vi "Omniax_mDrive_Xonly_2017APXNoBK.vi"() -> ()   [LabVIEW 2015]
uses:
  <vilib>/Utility/file.llb/Read From Spreadsheet File (I64).vi
  <vilib>/Instr/_visa.llb/VISA Configure Serial Port (Instr).vi
  <userlib>/caLab/Private/Get_PV.vi
  Omniax_mDrive_GNDGlobal.vi
  <userlib>/caLab/Private/Put_DBL_PV.vi
  <vilib>/Utility/file.llb/Write To Spreadsheet File (I64).vi
  <vilib>/Utility/file.llb/Read From Spreadsheet File (string).vi
  <vilib>/Utility/file.llb/Write To Spreadsheet File (DBL).vi
panel:
  out "read buffer":string
  in  "APX:MX_RQ":dbl min=-1.5 max=1.5
  in  "APX:MX_VLC_RQ":dbl min=0.0 max=0.1 step=0.01
  out "PR P":string
  in  "X Velocity SP step/sec":i32 min=1 max=12800
  in  "X Step SP":i32=-20000 min=-2304000 max=2304000 step=500
  out "X Step PV":i32 max=2000
  out "Boolean 2":bool
  out "R Velocity MVdeg/sec":dbl format="%.3f"
  out "R Position MV deg":dbl
  out "Z Velocity MV mm/sec":dbl format="%.3f"
  out "Z Position MV mm":dbl
  out "Y Velocity MV mm/sec":dbl format="%.3f"
  out "Y Position MV mm":dbl
  out "X Velocity MV mm/sec":dbl format="%.3f"
  out "X Position MV mm":dbl
  out "Presets":i32[][](array[numeric])
  in  "stop":bool
  in  "Tab Control 3":enum32{"Status", "Reset"}(tab)
  out "APX:X_LIM":bool
  out "APX:MX_MVG":bool
  out "APX:MX_RDY":bool
  out "sample NC":bool
  out "Z<350?":bool
  in  "Reset X Position mm":dbl
  out "Reset X Motor Steps":i32
  in  "Reset":bool
  out "R Backlash steps/sec":i32
  out "R Backlash":i32
  out "R Holding Current %":i32
  out "R Run Current %":i32
  out "R offset deg":dbl
  out "R deg/rev":dbl
  out "R steps/rev":u32
  out "R velocity PV step/sec":i32
  out "Z Backlash steps/sec":i32
  out "Z Backlash":i32
  out "Z Holding Current %":i32
  out "Z Run Current %":i32
  out "Z offset mm":dbl
  out "Z mm/rev":dbl
  out "Z steps/rev":u32
  out "Z  velocity PV step/sec":i32
  out "APX:MX_PV":dbl
  out "X velocity PV step/sec":i32
  out "X Backlash steps/sec":i32
  out "X Backlash":i32
  out "X Holding Current %":i32
  out "X Run Current %":i32
  out "X offset mm":dbl
  out "X mm/rev":dbl
  out "X steps/rev":u32
  out "X MAXPOS":i32=-34296
  out "X MINPOS":i32=-94296
  out "X COM PORT":refnum<visa-resource-name>="COM5"
  out "Y Backlash steps/sec":i32
  out "Y Backlash":i32
  out "Y Holding Current %":i32
  out "Y Run Current %":i32
  out "Y offset mm":dbl
  out "Y mm/rev":dbl
  out "Y steps/rev":u32
  out "Y velocity PV step/sec":i32
  in  "APX:MXYZR_STOP":bool
  # "APX:MX"
  # "Goto position"
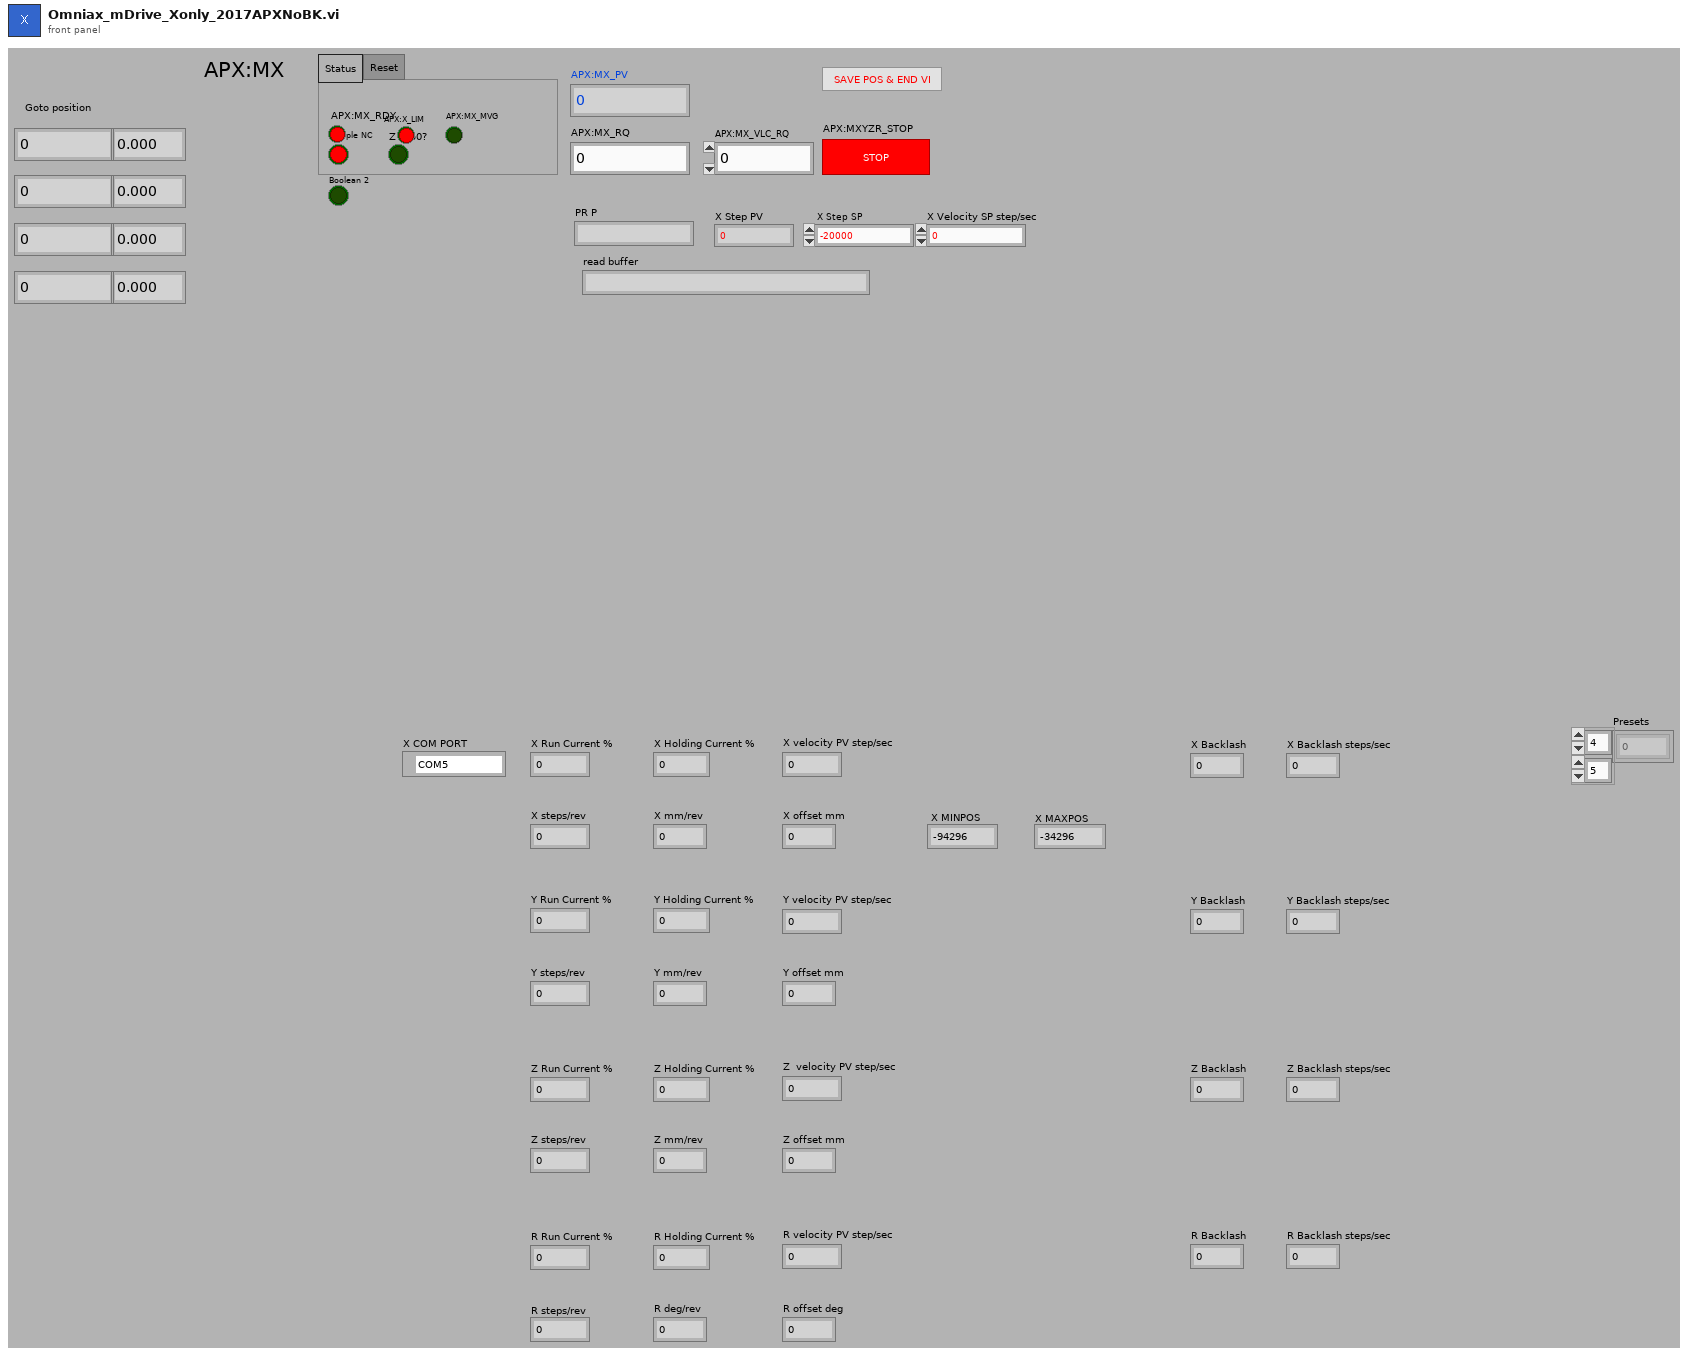
[diagram p1: front panel]
types:
  T1 = enum16{"Stop", "Reset", "Run Current", "Holding Current", "Accel Rate", "Decel Rate", "Move to Relative Position", "Move to Absolute Position", "Echo Mode", "Print Parameter", "Send String", "Microstep Resolution", "Set Current Position", "Max Velocity"}
  T2 = enum8{"Enabled", "Disabled", "Disabled and Grayed Out"}
  T3 = cluster{"first row[0]":i64, "first row[1]":i64, "first row[2]":i64, "first row[3]":i64, "first row[4]":i64, "first row[5]":i64, "first row[6]":i64, "first row[7]":i64, "first row[8]":i64}
  T4 = cluster{"Value[0]":i32, "Value[1]":i32, "Value[2]":i32, "Value[3]":i32, "Value[4]":i32, "Value[5]":i32, "Value[6]":i32, "Value[7]":i32, "Value[8]":i32}
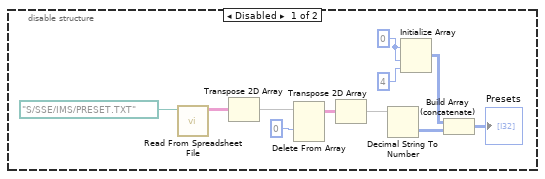
[diagram p2: hidden frame]
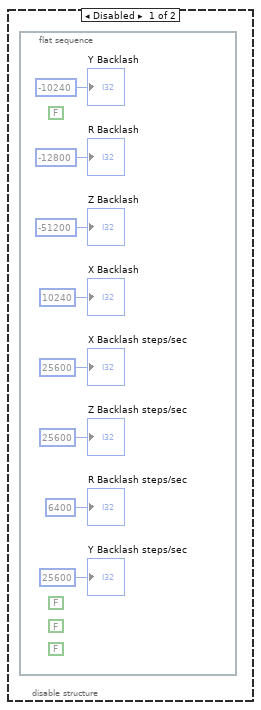
[diagram p3: hidden frame]
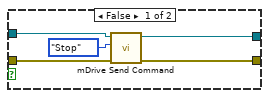
[diagram p9: hidden frame]
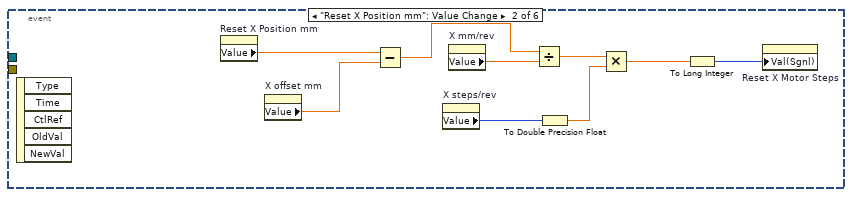
[diagram p14: hidden frame]
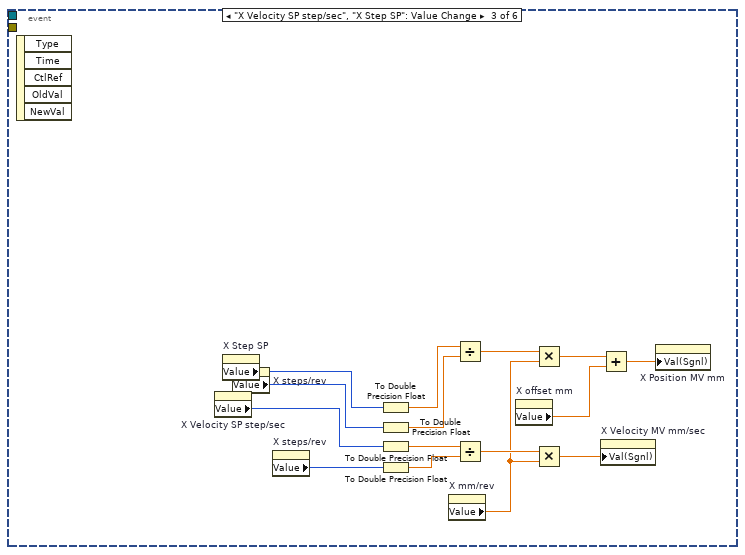
[diagram p15: hidden frame]
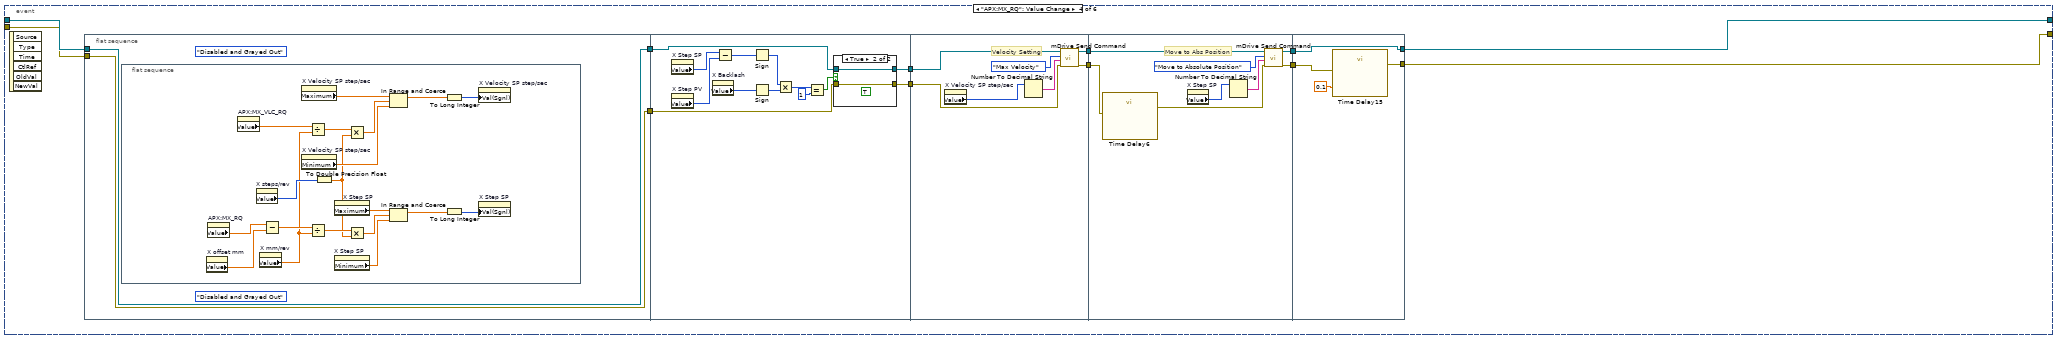
[diagram p16: hidden frame]
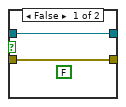
[diagram p17: hidden frame]
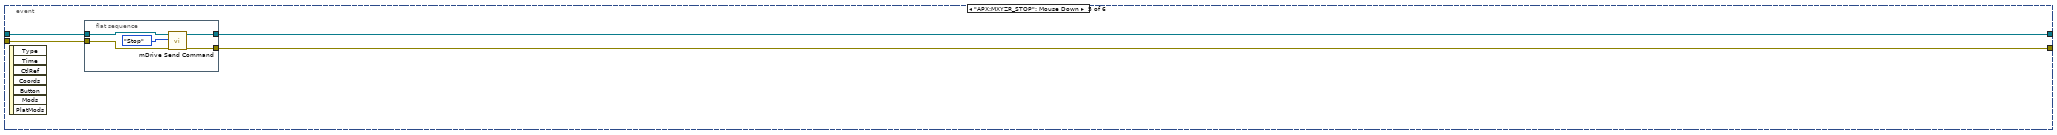
[diagram p18: hidden frame]
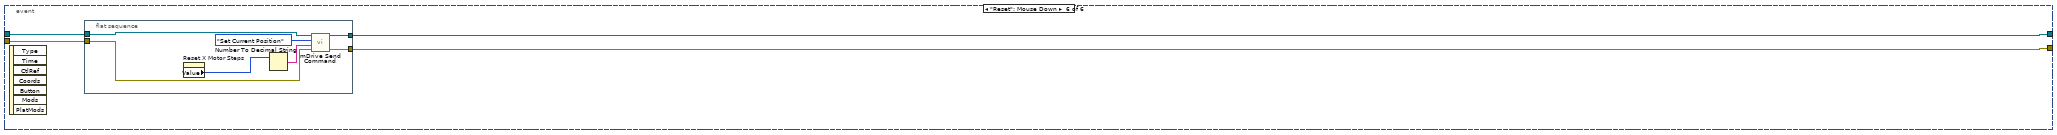
[diagram p19: hidden frame]
diagram:
  n1 = flat-sequence {
    tunnel: [w27] -> w9
    tunnel: [w26] -> w8
    tunnel: [w37] -> w12
    tunnel: w9 -> [w43]
    tunnel: w8 -> [w44]
    tunnel: [w38] -> w2
    tunnel: [w36] -> w1
    tunnel: w12 -> [_]
    tunnel: [w48] -> w11
    tunnel: [w51] -> w10
    tunnel: w2 -> [w49]
    tunnel: w1 -> [w47]
    tunnel: [w60] -> w25
    tunnel: [w62] -> w24
    tunnel: w11 -> [w61]
    tunnel: w10 -> [w63]
    tunnel: w25 -> [w70]
    tunnel: [w69] -> w23
    tunnel: w24 -> [w67]
    tunnel: [w68] -> w22
    tunnel: [w80] -> w21
    tunnel: [w81] -> w20
    tunnel: w23 -> [w79]
    tunnel: w22 -> [w78]
    tunnel: w21 -> [w91]
    tunnel: w20 -> [w90]
    tunnel: [w93] -> w15
    tunnel: [w92] -> w14
    tunnel: [w87] -> w13
    tunnel: [w98] -> w18
    tunnel: [w99] -> w19
    tunnel: w15 -> [w99]
    tunnel: w14 -> [w98]
    tunnel: w13 -> [w94]
    frame #0 {
      w34 = refnum<visa-resource-name> "COM12" ("COM PORT")
      w32 = u16 0 items=["None", "XON/XOFF", "RTS/CTS", "XON/XOFF & RTS/CTS", "DTR/DSR", "XON/XOFF & DTR/DSR"] ("flow control (0:none)")
      w31 = u16 10 items=["1.0"=10, "1.5"=15, "2.0"=20] ("stop bits (10: 1 bit)")
      # "Stop bits"
      n2 = call-poly "VISA Configure Serial Port"("VISA resource name"=w34, "timeout (10sec)"=u32 10000, "baud rate (9600)"=u32 9600, "data bits (8)"=u16 8, "parity (0:none)"=enum16{"None", "Odd", "Even", "Mark", "Space"}."None", "stop bits (10: 1 bit)"=w31, "flow control (0:none)"=w32) -> ("VISA resource name out"=w27:refnum<visa-resource-name>, "error out"=w26:errorcluster)  [unwired: 7 in]
      "X COM PORT" <- w34
    }
    frame #1 {
      n3 = VISA Flush I/O Buffer(VISA resource name=w43) -> (VISA resource name out=w42:refnum<visa-resource-name>)  [unwired: 2 in, 1 out]
      n4 = call "mDrive Send Command.vi"("error in (no error)"=w44, "Extra"="EM 2", "Command"=T1."Send String", "VISA resource name"=w42) -> ("error out"=w39:errorcluster, "VISA resource name out"=w37:refnum<visa-resource-name>)  [unwired: 3 in, 1 out]
      n5 = call "mDrive Send Command.vi"("error in (no error)"=w39, "Extra"="PR EE", "Command"=T1."Send String", "VISA resource name"=w37) -> ("error out"=w38:errorcluster, "read buffer"=→"read buffer":string, "VISA resource name out"=w36:refnum<visa-resource-name>)  [unwired: 3 in]
    }
    frame #2 {
      n6 = Number To Decimal String(number=1000000) -> (decimal integer string=w52:string)  [unwired: 1 in]
      n7 = call "mDrive Send Command.vi"("error in (no error)"=w49, "Extra"=w52, "Command"=T1."Accel Rate", "VISA resource name"=w47) -> ("error out"=w50:errorcluster, "VISA resource name out"=w56:refnum<visa-resource-name>)  [unwired: 3 in, 1 out]
      n8 = call "mDrive Send Command.vi"("error in (no error)"=w50, "Extra"=w52, "Command"=T1."Decel Rate", "VISA resource name"=w56) -> ("error out"=w51:errorcluster, "VISA resource name out"=w48:refnum<visa-resource-name>)  [unwired: 3 in, 1 out]
    }
    frame #3 {
      # "Run Current %"
      n9 = property on="X Run Current %" class="DigNum (strict)"() -> ("Value"=w58:i32)  [unwired: 2 in, 2 out]
      n10 = Number To Decimal String(number=w58) -> (decimal integer string=w59:string)  [unwired: 1 in]
      n11 = call "mDrive Send Command.vi"("error in (no error)"=w63, "Extra"=w59, "Command"=T1."Run Current", "VISA resource name"=w61) -> ("error out"=w62:errorcluster, "VISA resource name out"=w60:refnum<visa-resource-name>)  [unwired: 3 in, 1 out]
    }
    frame #4 {
      # "Holding Current %"
      n12 = property on="X Holding Current %" class="DigNum (strict)"() -> ("Value"=w65:i32)  [unwired: 2 in, 2 out]
      n13 = Number To Decimal String(number=w65) -> (decimal integer string=w66:string)  [unwired: 1 in]
      n14 = call "mDrive Send Command.vi"("error in (no error)"=w67, "Extra"=w66, "Command"=T1."Holding Current", "VISA resource name"=w70) -> ("error out"=w68:errorcluster, "VISA resource name out"=w69:refnum<visa-resource-name>)  [unwired: 3 in, 1 out]
    }
    frame #5 {
      # "Velocity Max"
      n15 = property on="X Velocity SP step/sec" class="DigNum (strict)"() -> ("Value"=w77:i32)  [unwired: 2 in, 2 out]
      n16 = Number To Decimal String(number=w77) -> (decimal integer string=w76:string)  [unwired: 1 in]
      n17 = call "mDrive Send Command.vi"("error in (no error)"=w78, "Extra"=w76, "Command"=T1."Max Velocity", "VISA resource name"=w79) -> ("error out"=w74:errorcluster, "VISA resource name out"=w84:refnum<visa-resource-name>)  [unwired: 3 in, 1 out]
      n18 = call "mDrive Send Command.vi"("error in (no error)"=w74, "Extra"="VM", "Command"=T1."Print Parameter", "VISA resource name"=w84) -> ("error out"=w81:errorcluster, "read buffer"=w82:string, "VISA resource name out"=w80:refnum<visa-resource-name>)  [unwired: 3 in]
      n19 = Decimal String To Number(string=w82, offset=0) -> (number=w75:i32)  [unwired: 1 in, 1 out]
      n20 = property on="X velocity PV step/sec" class="DigNum (strict)"("Val(Sgnl)"=w75) -> ()  [unwired: 2 in, 2 out]
    }
    frame #6 {
      # "PRINT POSITION"
      n21 = call "mDrive Send Command.vi"("error in (no error)"=w90, "Extra"="P", "Command"=T1."Print Parameter", "VISA resource name"=w91) -> ("error out"=w92:errorcluster, "read buffer"=w89:string, "VISA resource name out"=w93:refnum<visa-resource-name>)  [unwired: 3 in]
      n22 = Decimal String To Number(string=w89, offset=0) -> (number=w87:i32)  [unwired: 1 in, 1 out]
    }
    frame #7 {
      w96 = -2304000 ("lower limit")
      w97 = 2304000 ("upper limit")
      n23 = property on="X Step SP" class="DigNum (strict)"("Val(Sgnl)"=w94) -> ()  [unwired: 2 in, 2 out]
      n24 = property on="X Step SP" class="DigNum (strict)"("Maximum"=w97) -> ()  [unwired: 2 in, 2 out]
      n25 = In Range and Coerce(upper limit=w97, x=w94, lower limit=w96) -> (In Range?=w95:bool)  [unwired: 1 out]
      n26 = property on="X Step SP" class="DigNum (strict)"("Minimum"=w96) -> ()  [unwired: 2 in, 2 out]
      n27 = property on="APX:X_LIM" class="Bool (strict)"("Val(Sgnl)"=w95) -> ()  [unwired: 2 in, 2 out]
      "X MINPOS" <- w96
      "X MAXPOS" <- w97
    }
  }
  n28 = disable-structure shown="Enabled" {
    frame Disabled {
      w100 = 0 ("dimension size")
      n29 = call-poly <vilib>:"Read From Spreadsheet File.vi"("file path (dialog if empty)"=path "S:/SSE/IMS/PRESET.TXT") -> ("all rows"=w106:string[][])  [unwired: 6 in, 4 out]
      n30 = Transpose 2D Array(2D array=w106) -> (transposed array=w107:string[][])
      n31 = Delete From Array(array=w107, index (row)=0) -> (deleted portion=w108:string[], array with subset deleted=w110:string[][])  [unwired: 2 in]
      n32 = Transpose 2D Array(2D array=w110) -> (transposed array=w111:string[][])
      n33 = Decimal String To Number(string=w111) -> (number=w109:i32[][])  [unwired: 2 in, 1 out]
      n34 = Initialize Array(w100, w100, 4 ("dimension size")) -> (w103:i32[][])
      n35 = Build Array (concatenate)(w103, w109) -> (→"Presets":i32[][])
    }
    frame Enabled {
    }
  }
  n36 = flat-sequence {
    frame #0 {
      (unwired) 1.0 ("Data Entry Limits:Minimum")
      w115 = -3.0 ("R deg/rev")
      w113 = u32 51200 ("step/rev")
      n37 = To Double Precision Float(number=w113) -> (double precision float=w114:dbl)
      n38 = To Double Precision Float(number=10000 ("Value (Signaling)")) -> (double precision float=w119:dbl)
      n39 = Divide(x=w119, y=w114) -> (x/y=w118:dbl)
      n40 = Multiply(x=w118, y=w115) -> (x*y=w116:dbl)
      n41 = Absolute Value(x=w116) -> ()  [unwired: 1 out]
      "R offset deg" <- 0.0 ("R offset deg")
      "R deg/rev" <- w115
      "R steps/rev" <- w113
    }
  }
  n42 = flat-sequence {
    frame #0 {
      w121 = 0.2 ("Z mm/rev")
      w120 = u32 51200 ("step/rev")
      (unwired) 1.0 ("Data Entry Limits:Minimum")
      n43 = To Double Precision Float(number=204800 ("Value (Signaling)")) -> (double precision float=w125:dbl)
      n44 = To Double Precision Float(number=w120) -> (double precision float=w124:dbl)
      n45 = Divide(x=w125, y=w124) -> (x/y=w123:dbl)
      n46 = Multiply(x=w123, y=w121) -> ()  [unwired: 1 out]
      "Z offset mm" <- 0.0 ("Z offset mm")
      "Z mm/rev" <- w121
      "Z steps/rev" <- w120
    }
  }
  n47 = disable-structure shown="Enabled" {
    frame Disabled {
      n48 = flat-sequence {
        frame #0 {
          w127 = FALSE ("Value (Signaling)")
          w130 = FALSE ("Value (Signaling)")
          w133 = FALSE ("Value (Signaling)")
          w134 = FALSE ("Value (Signaling)")
          "Z Backlash steps/sec" <- 25600 ("Z Backlash steps/sec")
          "Z Backlash" <- -51200 ("Z Backlash")
          "X Backlash steps/sec" <- 25600 ("Value (Signaling)")
          "X Backlash" <- 10240 ("Backlash2")
          "Y Backlash" <- -10240 ("Backlash2")
          "Y Backlash steps/sec" <- 25600 ("Value (Signaling)")
          "R Backlash steps/sec" <- 6400 ("R Backlash steps/sec")
          "R Backlash" <- -12800 ("R Backlash")
        }
      }
    }
    frame Enabled {
    }
  }
  n49 = flat-sequence {
    frame #0 {
      "Z Holding Current %" <- 20 ("Z Holding Current %")
      "Z Run Current %" <- 40 ("Z Run Current %")
      "X Run Current %" <- 40 ("Run Current %")
      "X Holding Current %" <- 20 ("Holding Current %")
      "Y Run Current %" <- 40 ("Run Current %")
      "Y Holding Current %" <- 20 ("Holding Current %")
      "R Holding Current %" <- 15 ("R Holding Current %")
      "R Run Current %" <- 80 ("R Run Current %")
    }
  }
  n50 = flat-sequence {
    frame #0 {
      (unwired) 0.1 ("Value (Signaling)")
      (unwired) FALSE ("Value (Signaling)")
      (unwired) T2."Disabled and Grayed Out" ("Disabled")
      (unwired) T2."Disabled and Grayed Out" ("Disabled")
      (unwired) 0.1 ("Value (Signaling)")
      (unwired) FALSE ("Value (Signaling)")
      (unwired) 0.1 ("Value (Signaling)")
      (unwired) FALSE ("Value (Signaling)")
      (unwired) 0.1 ("Value (Signaling)")
      (unwired) FALSE ("Value (Signaling)")
    }
  }
  n51 = flat-sequence {
    frame #0 {
      w149 = 0.2 ("MM/rev")
      w152 = u32 51200 ("step/rev")
      w147 = 12800 ("Value (Signaling)")
      # "a=1000000"
      n52 = property on="X Velocity SP step/sec" class="DigNum (strict)"("Minimum"=1.0 ("Data Entry Limits:Minimum")) -> ()  [unwired: 2 in, 2 out]
      n53 = To Double Precision Float(number=w147) -> (double precision float=w153:dbl)
      n54 = To Double Precision Float(number=w152) -> (double precision float=w151:dbl)
      n55 = property on="X Velocity SP step/sec" class="DigNum (strict)"("Val(Sgnl)"=w147) -> ()  [unwired: 2 in, 2 out]
      n56 = property on="X Velocity SP step/sec" class="DigNum (strict)"("Maximum"=w153) -> ()  [unwired: 2 in, 2 out]
      n57 = Divide(x=w153, y=w151) -> (x/y=w148:dbl)
      n58 = Multiply(x=w148, y=w149) -> (x*y=w150:dbl)
      n59 = property on="APX:MX_VLC_RQ" class="DigNum (strict)"("Val(Sgnl)"=w150) -> ()  [unwired: 2 in, 2 out]
      "X offset mm" <- 0.0 ("offset")
      "X steps/rev" <- w152
      "X mm/rev" <- w149
    }
  }
  n60 = flat-sequence {
    frame #0 {
      w158 = 0.2 ("MM/rev")
      w160 = u32 51200 ("step/rev")
      (unwired) 1.0 ("Data Entry Limits:Minimum")
      n61 = To Double Precision Float(number=128000 ("Value (Signaling)")) -> (double precision float=w161:dbl)
      n62 = To Double Precision Float(number=w160) -> (double precision float=w159:dbl)
      n63 = Divide(x=w161, y=w159) -> (x/y=w157:dbl)
      n64 = Multiply(x=w157, y=w158) -> ()  [unwired: 1 out]
      "Y offset mm" <- 0.0 ("offset")
      "Y steps/rev" <- w160
      "Y mm/rev" <- w158
    }
  }
  n65 = call-poly <vilib>:"Read From Spreadsheet File.vi"("file path (dialog if empty)"=path "S:/SSE/IMS/POSX.TXT") -> ("first row"=w6:i64[])  [unwired: 6 in, 4 out]
  n66 = Array To Cluster(array=w6) -> (cluster=w5:T3)
  n67 = Unbundle(w5) -> ("first row[0]"=w3:i64)  [unwired: 8 out]
  n68 = property on="Reset X Motor Steps" class="DigNum (strict)"("Val(Sgnl)"=w3) -> ()  [unwired: 2 in, 2 out]
  n69 = while {
    tunnel: w19 -> [w167]
    tunnel: w18 -> [w166]
    tunnel: [w165] -> w17
    tunnel: [w164] -> w16
    stop <- "stop" stop-if-true
    n70 = disable-structure shown="Disabled" {
      frame Disabled {
        n71 = case shown="True" {
          selector: _ -> [_ _]
          tunnel: _ -> [_ w194]
          frame False {
          }
          frame True {
            n72 = property on="Presets" class="Arr (strict)"() -> ("Value"=w191:i32[][])  [unwired: 2 in, 2 out]
            n73 = Index Array(array=w191, index (row)=w194) -> (element=w193:i32[])  [unwired: 1 in]
            n74 = Array To Cluster(array=w193) -> (cluster=w192:T4)
            n75 = Unbundle(w192) -> ("Value[0]"=w190:i32, "Value[1]"=w189:i32, "Value[2]"=w188:i32, "Value[3]"=w187:i32)  [unwired: 5 out]
            n76 = property on="X Step SP" class="DigNum (strict)"("Val(Sgnl)"=w190) -> ()  [unwired: 2 in, 2 out]
          }
        }
        n77 = case shown="True" w170 {
          tunnel: [_ w186] -> w171
          frame False {
          }
          frame True {
            n78 = property on="X Step PV" class="DigNum (strict)"() -> ("Value"=w181:i32)  [unwired: 2 in, 2 out]
            n79 = Build Array(w186) -> (w185:void[], w182:dbl)
            n80 = Build Array(w181) -> (w184:i32[], w180:i32, w179:i32, w178:i32)
            n81 = property on="Presets" class="Arr (strict)"() -> ("Value"=w183:i32[][])  [unwired: 2 in, 2 out]
            n82 = Build Array (concatenate)(w183, w184) -> (w177:i32[][])
            n83 = property on="Presets" class="Arr (strict)"("Val(Sgnl)"=w177) -> ()  [unwired: 2 in, 2 out]
          }
        }
        n84 = case shown="True" w169 {
          tunnel: w171 -> [_ w176]
          frame False {
          }
          frame True {
            n85 = Delete From Array(array=w176) -> (array with subset deleted=w175, index=w174:i32)  [unwired: 1 in, 1 out]
            n86 = property on="Presets" class="Arr (strict)"() -> ("Value"=w173:i32[][])  [unwired: 2 in, 2 out]
            n87 = Delete From Array(array=w173, index (row)=w174) -> (array with subset deleted=w172:i32[][])  [unwired: 2 in, 1 out]
            n88 = property on="Presets" class="Arr (strict)"("Val(Sgnl)"=w172) -> ()  [unwired: 2 in, 2 out]
          }
        }
      }
      frame Enabled {
      }
    }
    n89 = event shown="[0] Timeout" {
      selector: _ -> [_ _ _ _ _ _]
      dyn-events: _ -> [_ _ _ _ _ _]
      timeout: 100 -> [_ _ _ _ _ _]
      tunnel: w167 -> [w207 _ _ w393 w460 w471]
      tunnel: w166 -> [w205 _ _ w392 w459 w470]
      tunnel: [w209 _ _ w391 w462 w469] -> w165
      tunnel: [w208 _ _ w390 w461 w468] -> w164
      event Timeout {
        n90 = event-data() -> ()  [unwired: 1 in, 2 out]
        n91 = flat-sequence {
          tunnel: [w265] -> w220
          tunnel: [w243] -> w219
          tunnel: [w254] -> w218
          tunnel: [w234] -> w217
          tunnel: w206 -> [w233]
          tunnel: w204 -> [w232]
          tunnel: [w228] -> w203
          tunnel: w220 -> [w277]
          tunnel: [w277] -> w216
          tunnel: w219 -> [w276]
          tunnel: [w276] -> w215
          tunnel: w218 -> [w275]
          tunnel: [w275] -> w214
          tunnel: w217 -> [w274]
          tunnel: [w274] -> w213
          tunnel: w203 -> [w273]
          tunnel: [w273] -> w201
          tunnel: w216 -> [w281]
          tunnel: [w282] -> w212
          tunnel: w215 -> [w284]
          tunnel: [w283] -> w211
          tunnel: w214 -> [w280]
          tunnel: [w279] -> w210
          tunnel: w213 -> [w279]
          tunnel: [w278] -> w202
          tunnel: w201 -> [w278]
          tunnel: w212 -> [w296]
          tunnel: w211 -> [w297]
          tunnel: w210 -> [w298]
          tunnel: [w295] -> w208
          tunnel: [w294] -> w209
          tunnel: w202 -> [w292]
          frame #0 {
            w238 = 0.1 ("Delay Time (s)")
            n92 = call "mDrive Send Command.vi"("error in (no error)"=w232, "Extra"="P", "Command"=T1."Print Parameter", "VISA resource name"=w233) -> ("error out"=w260:errorcluster, "read buffer"=w264:string, "VISA resource name out"=w262:refnum<visa-resource-name>)  [unwired: 3 in]
            "PR P" <- w264
            n93 = call "Time Delay12"("error in (no error)"=w260, "Delay Time (s)"=w238) -> ("error out"=w259:errorcluster)  [unwired: 9 in]
            n94 = Decimal String To Number(string=w264, offset=0) -> (number=w245:i32)  [unwired: 1 in, 1 out]
            n95 = property on="X Step SP" class="DigNum (strict)"() -> ("Maximum"=w256:dbl)  [unwired: 2 in, 2 out]
            n96 = property on="X Step SP" class="DigNum (strict)"() -> ("Minimum"=w258:dbl)  [unwired: 2 in, 2 out]
            n97 = To Long Integer(number=w245) -> (32bit integer=w246:i32)
            n98 = property on="X steps/rev" class="DigNum (strict)"() -> ("Value"=w252:u32)  [unwired: 2 in, 2 out]
            n99 = property on="X Step PV" class="DigNum (strict)"("Val(Sgnl)"=w246) -> ()  [unwired: 2 in, 2 out]
            n100 = disable-structure shown="Disabled" {
              disable-tunnel: [w272 _] -> w265
              disable-tunnel: w262 -> [w271 _]
              disable-tunnel: [w270 _] -> w261
              disable-tunnel: w259 -> [w269 _]
              disable-tunnel: T1."Print Parameter" ("Command") -> [w268 _]
              disable-tunnel: "MV" ("Extra") -> [w267 _]
              disable-tunnel: [w266 _] -> w231
              frame Disabled {
                n101 = call "mDrive Send Command.vi"("error in (no error)"=w269, "Extra"=w267, "Command"=w268, "VISA resource name"=w271) -> ("error out"=w270:errorcluster, "read buffer"=w266:string, "VISA resource name out"=w272:refnum<visa-resource-name>)  [unwired: 3 in]
              }
              frame Enabled {
              }
            }
            n102 = To Long Integer(number=w256) -> (32bit integer=w255:i32)
            n103 = To Long Integer(number=w258) -> (32bit integer=w257:i32)
            n104 = In Range and Coerce(upper limit=w255, x=w246, lower limit=w257) -> (In Range?=w254:bool)  [unwired: 1 out]
            n105 = To Double Precision Float(number=w246) -> (double precision float=w247:dbl)
            n106 = To Double Precision Float(number=w252) -> (double precision float=w253:dbl)
            n107 = property on="APX:X_LIM" class="Bool (strict)"("Val(Sgnl)"=w254) -> ()  [unwired: 2 in, 2 out]
            n108 = Divide(x=w247, y=w253) -> (x/y=w251:dbl)
            n109 = call "Time Delay11"("error in (no error)"=w261, "Delay Time (s)"=w238) -> ("error out"=w243:errorcluster)  [unwired: 9 in]
            n110 = Decimal String To Number(string=w231, offset=0 ("offset (0)")) -> (number=w237:i32)  [unwired: 1 in, 1 out]
            n111 = Not Equal?(x=w231, y="") -> (x != y?=w229:bool)
            n112 = property on="X mm/rev" class="DigNum (strict)"() -> ("Value"=w250:dbl)  [unwired: 2 in, 2 out]
            n113 = property on="X offset mm" class="DigNum (strict)"() -> ("Value"=w248:dbl)  [unwired: 2 in, 2 out]
            n114 = Multiply(x=w251, y=w250) -> (x*y=w249:dbl)
            n115 = Number To Boolean Array(number=w237) -> (Boolean array=w236:bool[])
            n116 = property on="APX:MX_RDY" class="Bool (strict)"("Val(Sgnl)"=w229) -> ()  [unwired: 2 in, 2 out]
            n117 = Add(x=w249, y=w248) -> (x+y=w228:dbl)
            n118 = Index Array(array=w236, index=0) -> (element=w234:bool)
            n119 = property on="APX:MX_PV" class="DigNum (strict)"("Val(Sgnl)"=w228) -> ()  [unwired: 2 in, 2 out]
            n120 = property on="APX:MX_MVG" class="Bool (strict)"("Val(Sgnl)"=w234) -> ()  [unwired: 2 in, 2 out]
          }
          frame #1 {
          }
          frame #2 {
            n121 = case shown="False" w280 {
              tunnel: w281 -> [w287 w291]
              tunnel: [w288 w291] -> w282
              tunnel: [w289 w290] -> w283
              tunnel: w284 -> [w286 w290]
              frame False {
                n122 = call "mDrive Send Command.vi"("error in (no error)"=w286, "Command"=T1."Stop", "VISA resource name"=w287) -> ("error out"=w289:errorcluster, "VISA resource name out"=w288:refnum<visa-resource-name>)  [unwired: 4 in, 1 out]
              }
              frame True {
              }
            }
            "Boolean 2" <- w280
          }
          frame #3 {
            n123 = disable-structure shown="Disabled" {
              disable-tunnel: w298 -> [w304 _]
              disable-tunnel: w297 -> [w302 _]
              disable-tunnel: w296 -> [w301 _]
              disable-tunnel: [w300 _] -> w295
              disable-tunnel: [w299 _] -> w294
              frame Disabled {
                n124 = Implies(1:w304) -> (0:w303:bool, 2:w305:bool)
                n125 = case shown="False" w303 {
                  tunnel: w302 -> [w312 w364]
                  tunnel: w301 -> [w311 w365]
                  tunnel: [w310 w364] -> w300
                  tunnel: [w309 w365] -> w299
                  frame False {
                    # "Backlash"
                    n126 = flat-sequence {
                      tunnel: [w327] -> w324
                      tunnel: [w329] -> w323
                      tunnel: [w328] -> w322
                      tunnel: w312 -> [w326]
                      tunnel: w311 -> [w325]
                      tunnel: w324 -> [w337]
                      tunnel: [w337] -> w321
                      tunnel: w323 -> [w336]
                      tunnel: w322 -> [w335]
                      tunnel: [w334] -> w320
                      tunnel: [w333] -> w319
                      tunnel: [w332] -> w308
                      tunnel: w321 -> [w347]
                      tunnel: w320 -> [w346]
                      tunnel: w319 -> [w344]
                      tunnel: [w345] -> w318
                      tunnel: [w344] -> w317
                      tunnel: [w343] -> w314
                      tunnel: [w342] -> w313
                      tunnel: w308 -> [w342]
                      tunnel: w318 -> [w358]
                      tunnel: w317 -> [w351]
                      tunnel: [w358] -> w316
                      tunnel: [w357] -> w315
                      tunnel: w314 -> [w357]
                      tunnel: w313 -> [w353]
                      tunnel: [w352] -> w306
                      tunnel: w316 -> [w362]
                      tunnel: w315 -> [w361]
                      tunnel: [w360] -> w310
                      tunnel: [w359] -> w307
                      tunnel: w306 -> [w359]
                      tunnel: [w363] -> w309
                      tunnel: w307 -> [w363]
                      frame #0 {
                        n127 = property on="X Backlash steps/sec" class="DigNum (strict)"() -> ("Value"=w327:i32)  [unwired: 2 in, 2 out]
                        n128 = Number To Decimal String(number=w327) -> (decimal integer string=w330:string)  [unwired: 1 in]
                        n129 = call "mDrive Send Command.vi"("error in (no error)"=w326, "Extra"=w330, "Command"=T1."Max Velocity", "VISA resource name"=w325) -> ("error out"=w328:errorcluster, "VISA resource name out"=w329:refnum<visa-resource-name>)  [unwired: 3 in, 1 out]
                      }
                      frame #1 {
                        n130 = property on="X Backlash" class="DigNum (strict)"() -> ("Value"=w332:i32)  [unwired: 2 in, 2 out]
                        n131 = Number To Decimal String(number=w332) -> (decimal integer string=w338:string)  [unwired: 1 in]
                        n132 = call "mDrive Send Command.vi"("error in (no error)"=w335, "Extra"=w338, "Command"=T1."Move to Relative Position", "VISA resource name"=w336) -> ("error out"=w334:errorcluster, "VISA resource name out"=w333:refnum<visa-resource-name>)  [unwired: 3 in, 1 out]
                      }
                      frame #2 {
                        n133 = To Double Precision Float(number=w342) -> (double precision float=w340:dbl)
                        n134 = To Double Precision Float(number=w347) -> (double precision float=w349:dbl)
                        n135 = Absolute Value(x=w340) -> (abs(x)=w341:dbl)
                        n136 = Divide(x=w341, y=w349) -> (x/y=w350:dbl)
                        n137 = Add(x=w350, y=0.3) -> (x+y=w343:dbl)
                        n138 = call "Time Delay13"("error in (no error)"=w346, "Delay Time (s)"=w343) -> ("error out"=w345:errorcluster)  [unwired: 9 in]
                      }
                      frame #3 {
                        n139 = Negate(x=w353) -> (-x=w354:i32)
                        n140 = Number To Decimal String(number=w354) -> (decimal integer string=w355:string)  [unwired: 1 in]
                        n141 = call "mDrive Send Command.vi"("Extra"=w355, "Command"=T1."Move to Relative Position", "VISA resource name"=w351) -> ("VISA resource name out"=w352:refnum<visa-resource-name>)  [unwired: 4 in, 2 out]
                      }
                      frame #4 {
                        n142 = call "Time Delay14"("error in (no error)"=w362, "Delay Time (s)"=w361) -> ("error out"=w360:errorcluster)  [unwired: 9 in]
                      }
                      frame #5 {
                        (unwired) FALSE ("Value (Signaling)")
                      }
                    }
                  }
                  frame True {
                  }
                }
              }
              frame Enabled {
              }
            }
            n143 = call-poly <userlib>:"CaLabPut.vi"("Value"=w292, "PV Name"="APX:OmniaxX") -> ()  [unwired: 6 in, 4 out]
          }
        }
        n144 = call-poly "CaLabGet.vi"("PV Name"="APX:OmniaxZ") -> ("1rst Value (number)"=w199:dbl)  [unwired: 8 in, 6 out]
        n145 = Less?(x=w199, y=349.0) -> (x < y?=w195:bool)
        "Z<350?" <- w195
        n146 = global read "Omniax_mDrive_GNDGlobal.vi" "sample NC"() -> (w197:bool)
        "sample NC" <- w197
        n147 = Or(x=w195, y=w197) -> (x .or. y?=w196:bool)
        n148 = case shown="True" w196 {
          tunnel: w207 -> [w225 w226]
          tunnel: w205 -> [w223 w227]
          tunnel: [w222 w227] -> w204
          tunnel: [w221 w226] -> w206
          frame False {
            n149 = call "mDrive Send Command.vi"("error in (no error)"=w223, "Command"=T1."Stop", "VISA resource name"=w225) -> ("error out"=w222:errorcluster, "VISA resource name out"=w221:refnum<visa-resource-name>)  [unwired: 4 in, 1 out]
          }
          frame True {
          }
        }
      }
      event "Reset X Position mm": Value Change {
        n150 = event-data() -> ()  [unwired: 1 in, 5 out]
        n151 = property on="Reset X Position mm" class="DigNum (strict)"() -> ("Value"=w374:dbl)  [unwired: 2 in, 2 out]
        n152 = property on="X offset mm" class="DigNum (strict)"() -> ("Value"=w366:dbl)  [unwired: 2 in, 2 out]
        n153 = Subtract(x=w374, y=w366) -> (x-y=w373:dbl)
        n154 = property on="X steps/rev" class="DigNum (strict)"() -> ("Value"=w368:u32)  [unwired: 2 in, 2 out]
        n155 = property on="X mm/rev" class="DigNum (strict)"() -> ("Value"=w367:dbl)  [unwired: 2 in, 2 out]
        n156 = Divide(x=w373, y=w367) -> (x/y=w372:dbl)
        n157 = To Double Precision Float(number=w368) -> (double precision float=w371:dbl)
        n158 = Multiply(x=w372, y=w371) -> (x*y=w370:dbl)
        n159 = To Long Integer(number=w370) -> (32bit integer=w369:i32)
        n160 = property on="Reset X Motor Steps" class="DigNum (strict)"("Val(Sgnl)"=w369) -> ()  [unwired: 2 in, 2 out]
      }
      event "X Velocity SP step/sec", "X Step SP": Value Change {
        n161 = event-data() -> ()  [unwired: 1 in, 5 out]
        n162 = property on="X Velocity SP step/sec" class="DigNum (strict)"() -> ("Value"=w386:i32)  [unwired: 2 in, 2 out]
        n163 = property on="X Step SP" class="DigNum (strict)"() -> ("Value"=w379:i32)  [unwired: 2 in, 2 out]
        n164 = property on="X steps/rev" class="DigNum (strict)"() -> ("Value"=w377:u32)  [unwired: 2 in, 2 out]
        n165 = property on="X steps/rev" class="DigNum (strict)"() -> ("Value"=w384:u32)  [unwired: 2 in, 2 out]
        n166 = To Double Precision Float(number=w379) -> (double precision float=w380:dbl)
        n167 = To Double Precision Float(number=w377) -> (double precision float=w383:dbl)
        n168 = To Double Precision Float(number=w386) -> (double precision float=w387:dbl)
        n169 = To Double Precision Float(number=w384) -> (double precision float=w389:dbl)
        n170 = property on="X mm/rev" class="DigNum (strict)"() -> ("Value"=w375:dbl)  [unwired: 2 in, 2 out]
        n171 = Divide(x=w380, y=w383) -> (x/y=w382:dbl)
        n172 = Divide(x=w387, y=w389) -> (x/y=w388:dbl)
        n173 = property on="X offset mm" class="DigNum (strict)"() -> ("Value"=w376:dbl)  [unwired: 2 in, 2 out]
        n174 = Multiply(x=w382, y=w375) -> (x*y=w381:dbl)
        n175 = Multiply(x=w388, y=w375) -> (x*y=w385:dbl)
        n176 = Add(x=w381, y=w376) -> (x+y=w378:dbl)
        n177 = property on="X Velocity MV mm/sec" class="DigNum (strict)"("Val(Sgnl)"=w385) -> ()  [unwired: 2 in, 2 out]
        n178 = property on="X Position MV mm" class="DigNum (strict)"("Val(Sgnl)"=w378) -> ()  [unwired: 2 in, 2 out]
      }
      event "APX:MX_RQ": Value Change {
        n179 = event-data() -> ()  [unwired: 1 in, 6 out]
        n180 = flat-sequence {
          tunnel: [w403] -> w395
          tunnel: [w402] -> w394
          tunnel: w393 -> [w403]
          tunnel: w392 -> [w402]
          tunnel: [w425] -> w397
          tunnel: [w424] -> w396
          tunnel: w395 -> [w427]
          tunnel: w394 -> [w426]
          tunnel: [w443] -> w399
          tunnel: [w442] -> w398
          tunnel: w397 -> [w441]
          tunnel: w396 -> [w440]
          tunnel: [w451] -> w401
          tunnel: [w450] -> w400
          tunnel: w399 -> [w449]
          tunnel: w398 -> [w448]
          tunnel: [w457] -> w390
          tunnel: [w458] -> w391
          tunnel: w401 -> [w458]
          tunnel: w400 -> [w456]
          frame #0 {
            (unwired) T2."Disabled and Grayed Out" ("Disabled")
            (unwired) T2."Disabled and Grayed Out" ("Disabled")
            n181 = flat-sequence {
              frame #0 {
                n182 = property on="X offset mm" class="DigNum (strict)"() -> ("Value"=w418:dbl)  [unwired: 2 in, 2 out]
                n183 = property on="APX:MX_RQ" class="DigNum (strict)"() -> ("Value"=w417:dbl)  [unwired: 2 in, 2 out]
                n184 = property on="APX:MX_VLC_RQ" class="DigNum (strict)"() -> ("Value"=w411:dbl)  [unwired: 2 in, 2 out]
                n185 = property on="X steps/rev" class="DigNum (strict)"() -> ("Value"=w420:u32)  [unwired: 2 in, 2 out]
                n186 = property on="X mm/rev" class="DigNum (strict)"() -> ("Value"=w404:dbl)  [unwired: 2 in, 2 out]
                n187 = Subtract(x=w417, y=w418) -> (x-y=w421:dbl)
                n188 = property on="X Velocity SP step/sec" class="DigNum (strict)"() -> ("Maximum"=w407:dbl)  [unwired: 2 in, 2 out]
                n189 = property on="X Velocity SP step/sec" class="DigNum (strict)"() -> ("Minimum"=w406:dbl)  [unwired: 2 in, 2 out]
                n190 = Divide(x=w411, y=w404) -> (x/y=w412:dbl)
                n191 = Divide(x=w421, y=w404) -> (x/y=w422:dbl)
                n192 = To Double Precision Float(number=w420) -> (double precision float=w405:dbl)
                n193 = property on="X Step SP" class="DigNum (strict)"() -> ("Maximum"=w414:dbl)  [unwired: 2 in, 2 out]
                n194 = property on="X Step SP" class="DigNum (strict)"() -> ("Minimum"=w413:dbl)  [unwired: 2 in, 2 out]
                n195 = Multiply(x=w412, y=w405) -> (x*y=w409:dbl)
                n196 = Multiply(x=w422, y=w405) -> (x*y=w416:dbl)
                n197 = In Range and Coerce(upper limit=w407, x=w409, lower limit=w406) -> (coerced(x)=w408:dbl)  [unwired: 1 out]
                n198 = In Range and Coerce(upper limit=w414, x=w416, lower limit=w413) -> (coerced(x)=w415:dbl)  [unwired: 1 out]
                n199 = To Long Integer(number=w408) -> (32bit integer=w410:i32)
                n200 = To Long Integer(number=w415) -> (32bit integer=w419:i32)
                n201 = property on="X Velocity SP step/sec" class="DigNum (strict)"("Val(Sgnl)"=w410) -> ()  [unwired: 2 in, 2 out]
                n202 = property on="X Step SP" class="DigNum (strict)"("Val(Sgnl)"=w419) -> ()  [unwired: 2 in, 2 out]
              }
            }
          }
          frame #1 {
            n203 = property on="X Step SP" class="DigNum (strict)"() -> ("Value"=w435:i32)  [unwired: 2 in, 2 out]
            n204 = property on="X Step PV" class="DigNum (strict)"() -> ("Value"=w434:i32)  [unwired: 2 in, 2 out]
            n205 = property on="X Backlash" class="DigNum (strict)"() -> ("Value"=w423:i32)  [unwired: 2 in, 2 out]
            n206 = Subtract(x=w435, y=w434) -> (x-y=w433:i32)
            n207 = Sign(1:w433) -> (0:w432:i32)
            n208 = Sign(1:w423) -> (0:w431:i32)
            n209 = Multiply(x=w432, y=w431) -> (x*y=w430:i32)
            n210 = Equal?(x=w430, y=1) -> (x = y?=w428:bool)
            n211 = case shown="True" w428 {
              tunnel: w427 -> [w437 w439]
              tunnel: w426 -> [w436 w438]
              tunnel: [w436 w438] -> w425
              tunnel: [w437 w439] -> w424
              frame False {
                (unwired) FALSE ("Value (Signaling)")
              }
              frame True {
                (unwired) TRUE ("Value (Signaling)")
              }
            }
          }
          frame #2 {
            # "Velocity Setting"
            n212 = property on="X Velocity SP step/sec" class="DigNum (strict)"() -> ("Value"=w444:i32)  [unwired: 2 in, 2 out]
            n213 = Number To Decimal String(number=w444) -> (decimal integer string=w445:string)  [unwired: 1 in]
            n214 = call "mDrive Send Command.vi"("error in (no error)"=w441, "Extra"=w445, "Command"=T1."Max Velocity", "VISA resource name"=w440) -> ("error out"=w442:errorcluster, "VISA resource name out"=w443:refnum<visa-resource-name>)  [unwired: 3 in, 1 out]
          }
          frame #3 {
            # "Move to Abs Position"
            n215 = call "Time Delay6"("error in (no error)"=w448) -> ("error out"=w447:errorcluster)  [unwired: 10 in]
            n216 = property on="X Step SP" class="DigNum (strict)"() -> ("Value"=w454:i32)  [unwired: 2 in, 2 out]
            n217 = Number To Decimal String(number=w454) -> (decimal integer string=w453:string)  [unwired: 1 in]
            n218 = call "mDrive Send Command.vi"("error in (no error)"=w447, "Extra"=w453, "Command"=T1."Move to Absolute Position", "VISA resource name"=w449) -> ("error out"=w450:errorcluster, "VISA resource name out"=w451:refnum<visa-resource-name>)  [unwired: 3 in, 1 out]
          }
          frame #4 {
            n219 = call "Time Delay15"("error in (no error)"=w456, "Delay Time (s)"=0.1) -> ("error out"=w457:errorcluster)  [unwired: 9 in]
          }
        }
      }
      event "APX:MXYZR_STOP": Mouse Down {
        n220 = event-data() -> ()  [unwired: 1 in, 7 out]
        n221 = flat-sequence {
          tunnel: [w466] -> w462
          tunnel: [w465] -> w461
          tunnel: w460 -> [w464]
          tunnel: w459 -> [w463]
          frame #0 {
            n222 = call "mDrive Send Command.vi"("error in (no error)"=w463, "Command"=T1."Stop", "VISA resource name"=w464) -> ("error out"=w465:errorcluster, "VISA resource name out"=w466:refnum<visa-resource-name>)  [unwired: 4 in, 1 out]
          }
        }
      }
      event "Reset": Mouse Down {
        n223 = event-data() -> ()  [unwired: 1 in, 7 out]
        n224 = flat-sequence {
          tunnel: [w472] -> w469
          tunnel: w470 -> [w475]
          tunnel: [w474] -> w468
          tunnel: w471 -> [w473]
          frame #0 {
            n225 = property on="Reset X Motor Steps" class="DigNum (strict)"() -> ("Value"=w476:i32)  [unwired: 2 in, 2 out]
            n226 = Number To Decimal String(number=w476) -> (decimal integer string=w477:string)  [unwired: 1 in]
            n227 = call "mDrive Send Command.vi"("error in (no error)"=w475, "Extra"=w477, "Command"=T1."Set Current Position", "VISA resource name"=w473) -> ("error out"=w474:errorcluster, "VISA resource name out"=w472:refnum<visa-resource-name>)  [unwired: 3 in, 1 out]
          }
        }
      }
    }
  }
  n228 = flat-sequence {
    tunnel: w17 -> [w485]
    tunnel: w16 -> [w483]
    tunnel: [w480] -> w7
    frame #0 {
      n229 = call "mDrive Send Command.vi"("error in (no error)"=w483, "Extra"="P", "Command"=T1."Print Parameter", "VISA resource name"=w485) -> ("error out"=w482:errorcluster, "read buffer"=w489:string, "VISA resource name out"=w484:refnum<visa-resource-name>)  [unwired: 3 in]
      n230 = call "Time Delay30"("error in (no error)"=w482) -> ("error out"=w479:errorcluster)  [unwired: 10 in]
      n231 = Decimal String To Number(string=w489, offset=0) -> (number=w481:i32)  [unwired: 1 in, 1 out]
      n232 = To Long Integer(number=w481) -> (32bit integer=w480:i32)
      n233 = call "mDrive Send Command.vi"("error in (no error)"=w479, "Command"=T1."Stop", "VISA resource name"=w484) -> ("error out"=w491:errorcluster, "VISA resource name out"=w492:refnum<visa-resource-name>)  [unwired: 4 in, 1 out]
      n234 = VISA Close(VISA resource name=w492, error in (no error)=w491) -> ()  [unwired: 1 out]
    }
  }
  n235 = flat-sequence {
    tunnel: w7 -> [w495]
    frame #0 {
      n236 = Build Array(w495) -> (w493:i32[])
      n237 = call-poly <vilib>:"Write To Spreadsheet File.vi"("1D data"=w493, "file path (dialog if empty)"=path "S:/SSE/IMS/POSX.TXT") -> ()  [unwired: 6 in, 1 out]
    }
    frame #1 {
      n238 = disable-structure shown="Disabled" {
        frame Disabled {
          n239 = property on="Presets" class="Arr (strict)"() -> ("Value"=w500:i32[][])  [unwired: 2 in, 2 out]
          n240 = Number To Decimal String(number=w500) -> (decimal integer string=w496:string[][])  [unwired: 1 in]
          n241 = Transpose 2D Array(2D array=w496) -> (transposed array=w497:string[][])
          n242 = Build Array(w497) -> ()  [unwired: 1 in, 1 out]
          n243 = Transpose 2D Array() -> (transposed array=w498:dbl[][])  [unwired: 1 in]
          n244 = call-poly <vilib>:"Write To Spreadsheet File.vi"("2D data"=w498, "file path (dialog if empty)"=path "S:/SSE/IMS/PRESETX.TXT") -> ()  [unwired: 6 in, 1 out]
        }
        frame Enabled {
        }
      }
    }
  }
